vi "dimension_detect.vi"(3 "input_machine_reference.lvclass":refnum<class "machine.lvclass">) -> (0 "SCPI_comand_array_size":u32, 1 "output_machine_reference.lvclass":refnum<class "machine.lvclass">)   [LabVIEW 2014, in "machine.lvclass"]
uses:
  machine.lvclass
  machine.lvclass/machine.ctl
  dll/SCPI_LUTs.dll
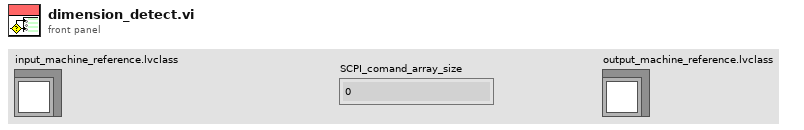
[diagram p1: front panel]
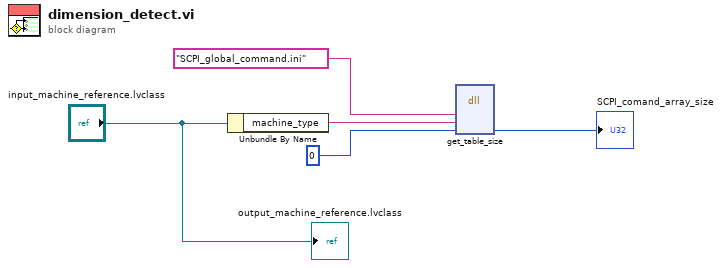
[diagram p0: block diagram]
diagram:
  n1 = Unbundle By Name("input_machine_reference.lvclass") -> ("machine_type"=w3:string)
  n2 = dll-call lib="C:/Users/DrippySummer/Documents/LabVIEW Data/SavaData/keithley_general_client/dll/SCPI_LUTs.dll" fn="get_table_size"("file_path"="SCPI_global_command.ini", "machine_type"=w3, "arr_size"=u32 0) -> ("arr_size"=→"SCPI_comand_array_size":u32)  [unwired: 6 in, 2 out]
  "output_machine_reference.lvclass" <- "input_machine_reference.lvclass"
